vi "setParameters.vi"(10 "Parameters":T1, 11 "ApplyAberrationByForcesCommand in":refnum<class "ApplyAberrationByForcesCommand.lvclass">) -> (3 "ApplyAberrationByForcesCommand out":refnum<class "ApplyAberrationByForcesCommand.lvclass">)   [LabVIEW 2016, in "ApplyAberrationByForcesCommand.lvclass"]
uses:
  ApplyAberrationByForcesCommand.lvclass
  DataTypes/Topics/CommandApplyAberrationByForces.ctl
  DataTypes/Topics/Parts/CommandId.ctl
  ApplyAberrationByForcesCommand.lvclass/ApplyAberrationByForcesCommand.ctl
  DataTypes/Topics/M1M3SupportTopics.lvlib
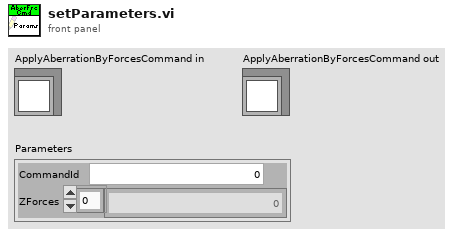
[diagram p1: front panel]
types:
  T1 = typedef "M1M3SupportTopics.lvlib/CommandApplyAberrationByForces.ctl" = cluster{"CommandId":T2, "ZForces":dbl[]}
  T2 = typedef "M1M3SupportTopics.lvlib/CommandId.ctl" = i32
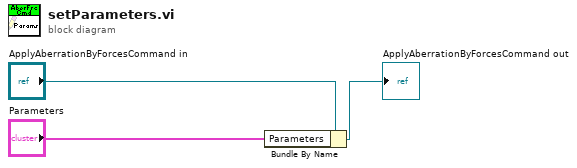
[diagram p0: block diagram]
diagram:
  n1 = Bundle By Name(cluster="ApplyAberrationByForcesCommand in", "Parameters"="Parameters") -> (→"ApplyAberrationByForcesCommand out":refnum<class "ApplyAberrationByForcesCommand.lvclass">)
